vi "Set_Channels_Map.vi"(3 "error in":errorcluster, 5 "Filename (.ini)":string="channels_map_default.ini") -> (0 "error out":errorcluster, 2 "Channels Map":T1)   [LabVIEW 2021]
uses:
  Channels_Map.ctl
  Channel_Cluster.ctl
  <vilib>/Utility/config.llb/Write Key (U32).vi
  <vilib>/Utility/config.llb/NI_LVConfig.lvlib
panel:
  in  "Reset map":bool
  in  "End configuration":bool
  in  "Remove channel":bool
  in  "Add channel":bool
  in  "Channel":u8=2 min=2 max=13 step=1
  in  "Channel name":string
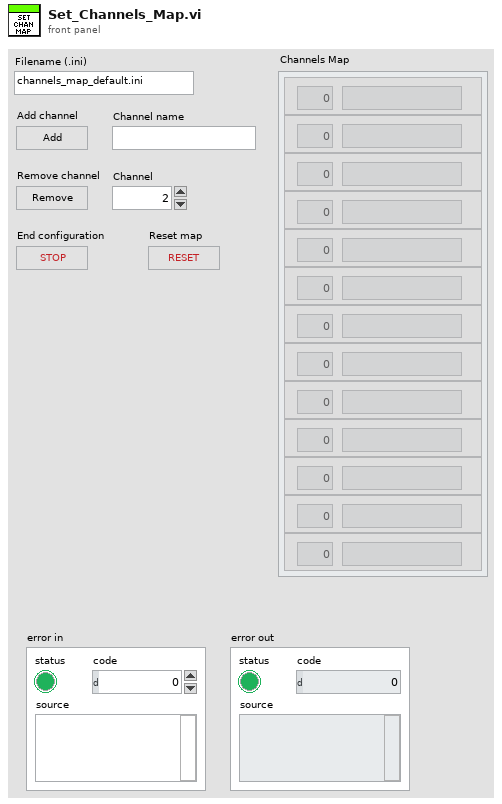
[diagram p1: front panel]
types:
  T1 = typedef "Channels_Map.ctl" = T2[]
  T2 = typedef "Channel_Cluster.ctl" = cluster{"Channel name":string, "Channel":u8}
  T3 = typedef "NI_LVConfig.lvlib/Config Data RefNum.ctl" = refnum<k1>
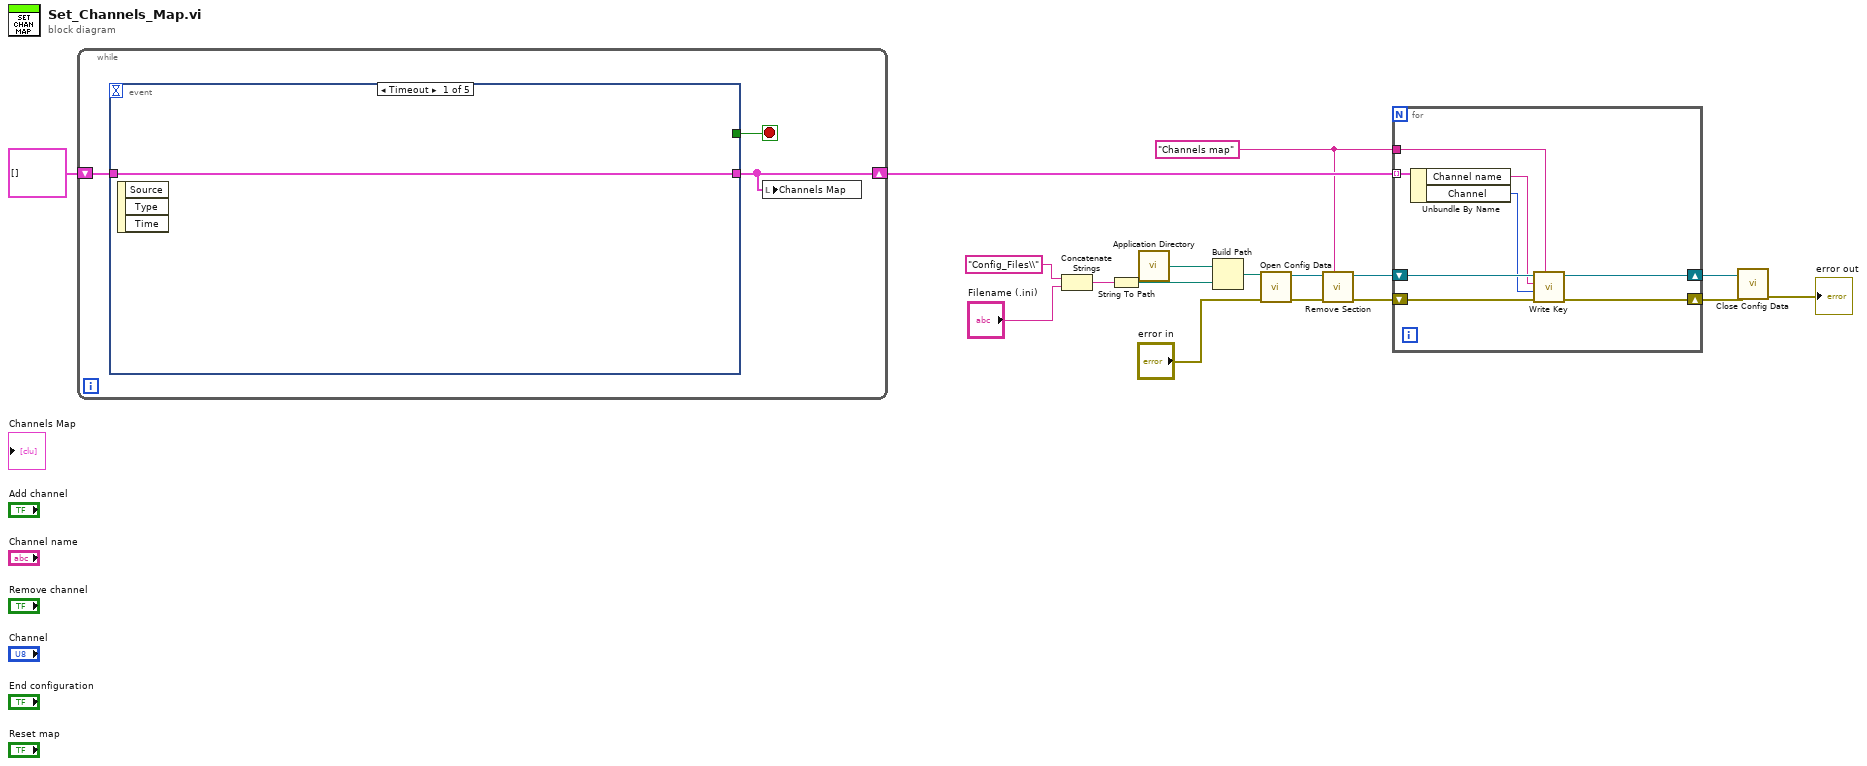
[diagram p0: block diagram]
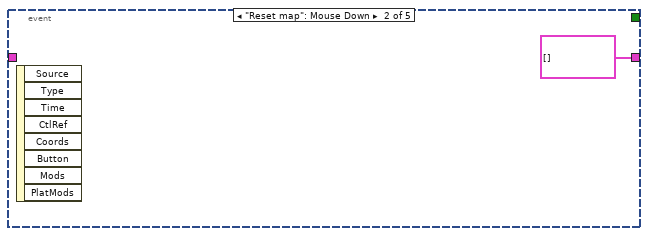
[diagram p2: hidden frame]
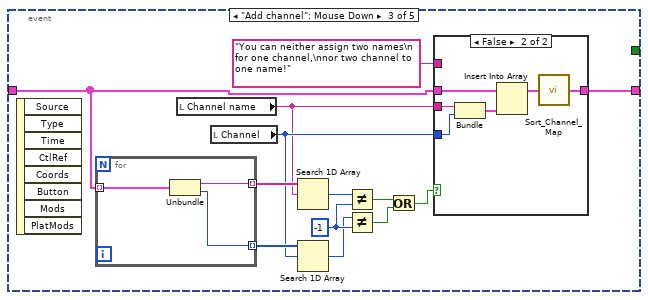
[diagram p3: hidden frame]
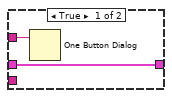
[diagram p4: hidden frame]
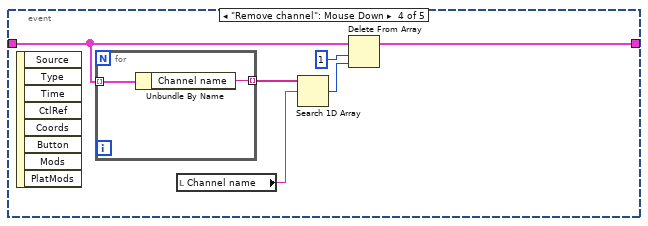
[diagram p5: hidden frame]
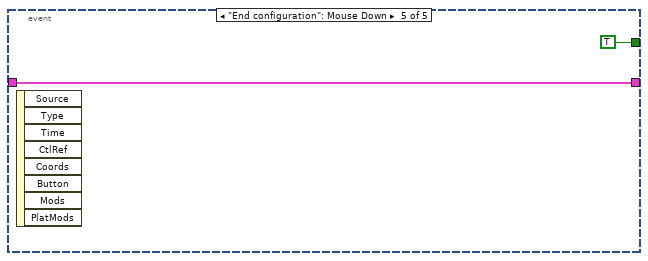
[diagram p6: hidden frame]
diagram:
  w5 = "Channels map" ("section")
  n1 = while {
    shift-right: [w19] -> w8
    shift-left: T1 [] ("Channels Map") -> [w20]
    stop <- w18 stop-if-true
    n2 = event shown="[0] Timeout" {
      selector: _ -> [_ _ _ _ _]
      dyn-events: _ -> [_ _ _ _ _]
      timeout: _ -> [_ _ _ _ _]
      tunnel: [w21 T1 [] ("Channels Map") w23 w47 w56] -> w19
      tunnel: w20 -> [w21 _ w25 w49 w56]
      tunnel: [_ _ _ _ TRUE] -> w18
      event Timeout {
        n3 = event-data() -> ()  [unwired: 1 in, 3 out]
      }
      event "Reset map": Mouse Down {
        n4 = event-data() -> ()  [unwired: 1 in, 8 out]
      }
      event "Add channel": Mouse Down {
        w33 = -1 ("y")
        n5 = event-data() -> ()  [unwired: 1 in, 8 out]
        n6 = for {
          tunnel: w25 -> [w46] mode=indexing
          tunnel: [w45] -> w29 mode=indexing
          tunnel: [w44] -> w30 mode=indexing
          n7 = Unbundle(w46) -> ("Channel name"=w44:string, "Channel"=w45:u8)
        }
        n8 = local read "Channel name"() -> (w26:string)
        n9 = local read "Channel"() -> (w27:u8)
        n10 = Search 1D Array(1D array=w30, element=w26) -> (index of element=w32:i32)  [unwired: 1 in]
        n11 = Search 1D Array(1D array=w29, element=w27) -> (index of element=w31:i32)  [unwired: 1 in]
        n12 = Not Equal?(x=w32, y=w33) -> (x != y?=w34:bool)
        n13 = Not Equal?(x=w31, y=w33) -> (x != y?=w35:bool)
        n14 = Or(x=w34, y=w35) -> (x .or. y?=w28:bool)
        n15 = case shown="False" w28 {
          tunnel: [w36 w38] -> w23
          tunnel: w25 -> [w36 w42]
          tunnel: w27 -> [_ w43]
          tunnel: "You can neither assign two names\n for one channel,\nnor two channel to one name!" ("message") -> [w37 _]
          tunnel: w26 -> [_ w40]
          frame True {
            n16 = One Button Dialog(message=w37) -> ()  [unwired: 1 in, 1 out]
          }
          frame False {
            n17 = Bundle("Channel name"=w40, "Channel"=w43) -> (w41:cluster{"Channel name":string, "Channel":u8})  [unwired: 1 in]
            n18 = Insert Into Array(array=w42, new element=w41) -> (w39:T1)  [unwired: 1 in]
            n19 = call "Sort_Channel_Map.vi"("Channels Map"=w39) -> ("Sorted Channels Map"=w38:T1)
          }
        }
      }
      event "Remove channel": Mouse Down {
        n20 = event-data() -> ()  [unwired: 1 in, 8 out]
        n21 = for {
          tunnel: w49 -> [w54] mode=indexing
          tunnel: [w53] -> w50 mode=indexing
          n22 = Unbundle By Name(w54) -> ("Channel name"=w53:string)
        }
        n23 = local read "Channel name"() -> (w48:string)
        n24 = Search 1D Array(1D array=w50, element=w48) -> (index of element=w52:i32)  [unwired: 1 in]
        n25 = Delete From Array(array=w49, length=1, index=w52) -> (array with subset deleted=w47:T1)  [unwired: 1 out]
      }
      event "End configuration": Mouse Down {
        n26 = event-data() -> ()  [unwired: 1 in, 8 out]
      }
    }
    n27 = local write "Channels Map"(w19) -> ()
  }
  n28 = Concatenate Strings("Config_Files\\" ("string"), "Filename (.ini)") -> (w16:string)
  n29 = String To Path(string=w16) -> (path=w13:path)
  n30 = call <vilib>:"Application Directory.vi"() -> ("Application Directory"=w10:path)
  n31 = Build Path(base path=w10, name or relative path=w13) -> (appended path=w11:path)
  n32 = call <vilib>:"Open Config Data.vi"("error in (no error)"="error in", "configuration file path"=w11) -> ("error out"=w2:errorcluster, "refnum"=w4:T3)  [unwired: 7 in, 1 out]
  n33 = call <vilib>:"Remove Section.vi"("section"=w5, "error in (no error)"=w2, "refnum"=w4) -> ("error out"=w1:errorcluster, "refnum out"=w3:T3)  [unwired: 6 in, 1 out]
  n34 = for {
    tunnel: w8 -> [w64] mode=indexing
    shift-right: [w59] -> w7
    shift-left: w3 -> [w62]
    shift-right: [w58] -> w6
    shift-left: w1 -> [w63]
    tunnel: w5 -> [w57]
    n35 = Unbundle By Name(w64) -> ("Channel name"=w60:string, "Channel"=w61:u8)
    n36 = call-poly <vilib>:"Write Key.vi"("section"=w57, "error in (no error)"=w63, "value"=w61, "key"=w60, "refnum"=w62) -> ("error out"=w58:errorcluster, "refnum out"=w59:T3)  [unwired: 4 in, 1 out]
  }
  n37 = call <vilib>:"Close Config Data.vi"("error in (no error)"=w6, "refnum"=w7) -> ("error out"=→"error out":errorcluster)  [unwired: 8 in, 1 out]
